vi "open_dev3.vi"(4 "ViStatus":T2, 7 "InterfaceInfo 2":T3) -> (0 "ViStatus 2":T2, 1 "drv_name":string, 2 "ModuleInfo":T1 {"DacScaleCoef" format="%#_2g"; "DacOffsetCoef" format="%#_2g"}, 3 "InterfaceInfo":T3)   [LabVIEW 2010]
uses:
  Rtusbapi.llb/3000pars.vi
  pdv_usb/wrRtusbapi.dll
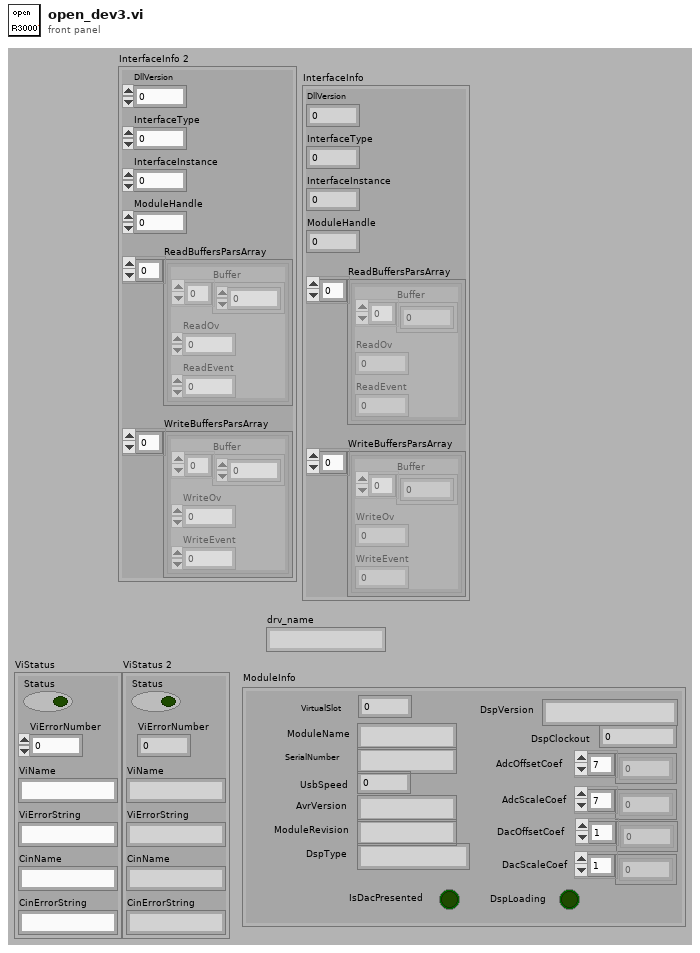
[diagram p1: front panel]
types:
  T1 = cluster{"VirtualSlot":u16, "ModuleName":string, "SerialNumber":string, "UsbSpeed":u8, "AvrVersion":string, "ModuleRevision":string, "DspType":string, "IsDacPresented":bool, "DspLoading":bool, "DspVersion":string, "DspClockout":u32, "AdcOffsetCoef":sgl[], "AdcScaleCoef":sgl[], "DacOffsetCoef":sgl[], "DacScaleCoef":sgl[]}
  T2 = cluster{"Status":bool, "ViErrorNumber":u32, "ViName":string, "ViErrorString":string, "CinName":string, "CinErrorString":string}
  T3 = cluster{"DllVersion":u32, "InterfaceType":u32, "InterfaceInstance":u32, "ModuleHandle":u32, "ReadBuffersParsArray":cluster{"Buffer":i16[], "ReadOv":u32, "ReadEvent":u32}[], "WriteBuffersParsArray":cluster{"Buffer":i16[], "WriteOv":u32, "WriteEvent":u32}[]}
  T4 = cluster{"CRC16":u16, "size":u16, "SerialNumber":string, "Name":string, "Revision":string, "DSPType":string, "IsDACPresent":u16, "DSPClockout":u32, "ADCOffset":sgl[], "ADCScale":sgl[], "DACOffset":sgl[], "DACScale":sgl[]}
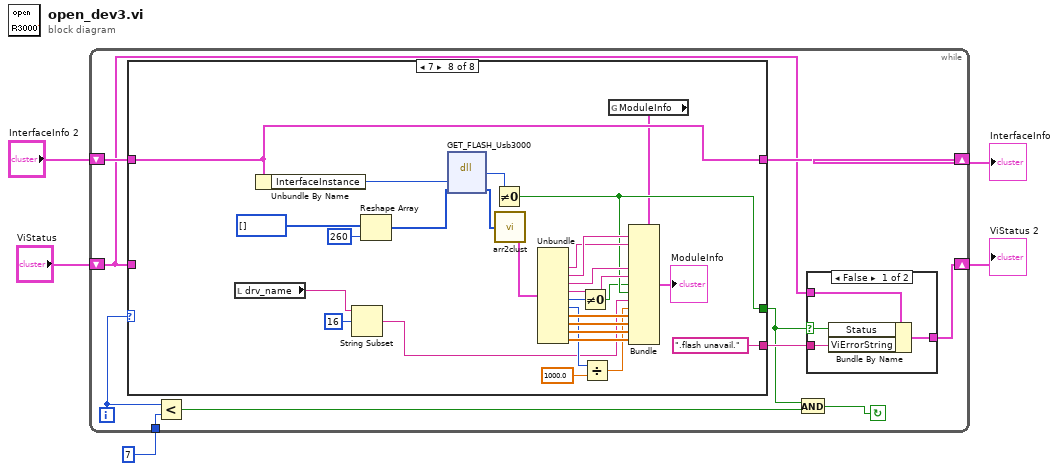
[diagram p0: block diagram]
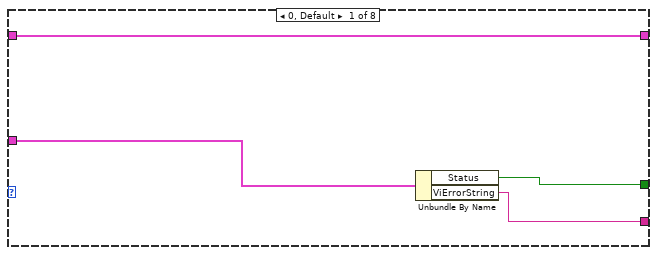
[diagram p3: hidden frame]
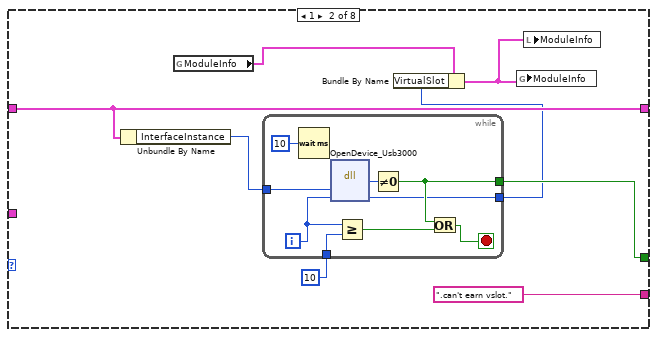
[diagram p4: hidden frame]
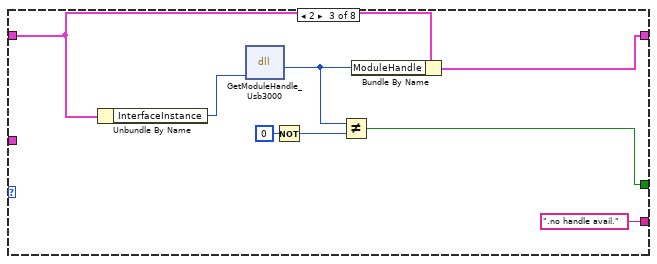
[diagram p5: hidden frame]
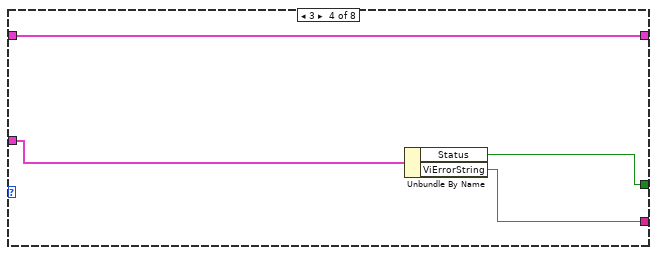
[diagram p6: hidden frame]
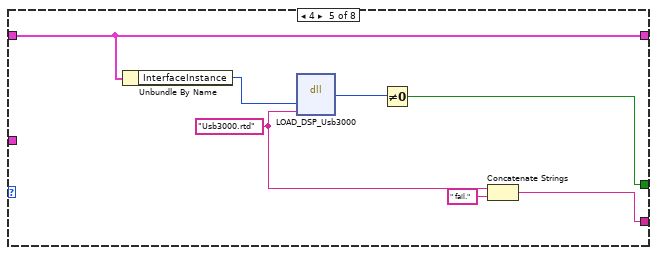
[diagram p7: hidden frame]
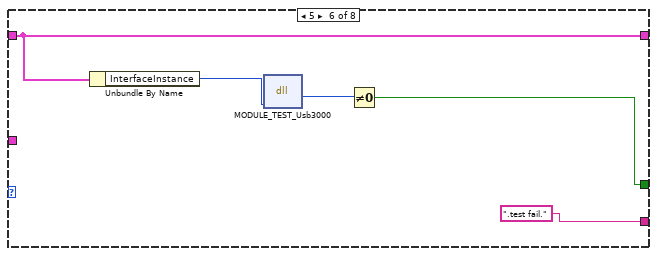
[diagram p8: hidden frame]
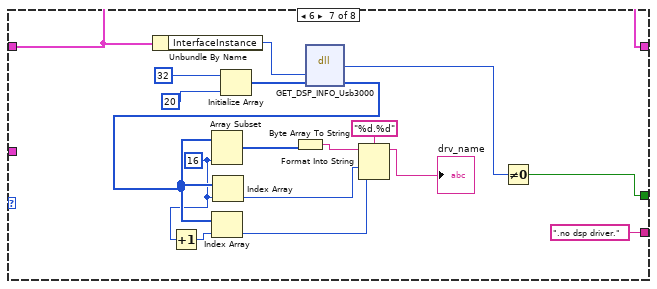
[diagram p9: hidden frame]
diagram:
  n1 = while {
    shift-right: [w14] -> w3
    shift-left: "InterfaceInfo 2" -> [w15]
    shift-right: [w12] -> w2
    shift-left: "ViStatus" -> [w13]
    tunnel: 7 ("y") -> [w6]
    i -> [w10]
    stop <- w7 continue-if-true
    n2 = case shown="7" w10 {
      tunnel: w15 -> [w24 w31 w48 w53 w60 w62 w79 w110]
      tunnel: [w24 w31 w47 w53 w60 w62 w79 w110] -> w14
      tunnel: w13 -> [w23 _ _ w51 _ _ _ _]
      tunnel: [w22 w30 w43 w52 w57 w63 w76 w96] -> w9
      tunnel: [w21 ".can't earn vslot." ("ViErrorString") ".no handle avail." ("ViErrorString") w50 w55 ".test fail." ("ViErrorString") ".no dsp driver." ("ViErrorString") ".flash unavail." ("ViErrorString")] -> w11
      frame 0, Default {
        n3 = Unbundle By Name(w23) -> ("Status"=w22:bool, "ViErrorString"=w21:string)
      }
      frame 1 {
        n4 = Unbundle By Name(w31) -> ("InterfaceInstance"=w32:u32)
        n5 = global read "3000pars.vi" "ModuleInfo"() -> (w26:T1)
        n6 = while {
          tunnel: w32 -> [w41]
          tunnel: [w37] -> w30
          tunnel: 10 -> [w38]
          tunnel: [w34] -> w27
          i -> [w39]
          stop <- w36 stop-if-true
          n7 = Wait (ms)(milliseconds to wait=u32 10) -> ()  [unwired: 1 out]
          n8 = dll-call lib="E:/Work/Andrew/Andrew_STEND/usb3k1064/pdv_usb/wrRtusbapi.dll" fn="OpenDevice_Usb3000"(w41, w39) -> (w40:i32, w34:u32)  [unwired: 4 in, 2 out]
          n9 = Greater Or Equal?(x=w39, y=w38) -> (x >= y?=w35:bool)
          n10 = Not Equal To 0?(x=w40) -> (x != 0?=w37:bool)
          n11 = Or(x=w37, y=w35) -> (x .or. y?=w36:bool)
        }
        n12 = Bundle By Name(cluster=w26, "VirtualSlot"=w27) -> (w25:T1)
        n13 = global write "3000pars.vi" "ModuleInfo"(w25) -> ()
        n14 = local write "ModuleInfo"(w25) -> ()
      }
      frame 2 {
        n15 = Unbundle By Name(w48) -> ("InterfaceInstance"=w49:u32)
        n16 = dll-call lib="E:/Work/Andrew/Andrew_STEND/usb3k1064/pdv_usb/wrRtusbapi.dll" fn="GetModuleHandle_Usb3000"(w49) -> (w46:u32)  [unwired: 4 in, 2 out]
        n17 = Not(x=u32 0 ("y")) -> (.not. x?=w44:u32)
        n18 = Not Equal?(x=w46, y=w44) -> (x != y?=w43:bool)
        n19 = Bundle By Name(cluster=w48, "ModuleHandle"=w46) -> (w47:T3)
      }
      frame 3 {
        n20 = Unbundle By Name(w51) -> ("Status"=w52:bool, "ViErrorString"=w50:string)
      }
      frame 4 {
        w56 = "Usb3000.rtd" ("input param")
        n21 = Unbundle By Name(w60) -> ("InterfaceInstance"=w59:u32)
        n22 = dll-call lib="E:/Work/Andrew/Andrew_STEND/usb3k1064/pdv_usb/wrRtusbapi.dll" fn="LOAD_DSP_Usb3000"(w59, w56) -> (w58:i32)  [unwired: 5 in, 2 out]
        n23 = Not Equal To 0?(x=w58) -> (x != 0?=w57:bool)
        n24 = Concatenate Strings(w56, " fail." ("string")) -> (w55:string)
      }
      frame 5 {
        n25 = Unbundle By Name(w62) -> ("InterfaceInstance"=w65:u32)
        n26 = dll-call lib="E:/Work/Andrew/Andrew_STEND/usb3k1064/pdv_usb/wrRtusbapi.dll" fn="MODULE_TEST_Usb3000"(w65) -> (w64:i32)  [unwired: 4 in, 2 out]
        n27 = Not Equal To 0?(x=w64) -> (x != 0?=w63:bool)
      }
      frame 6 {
        w66 = 16 ("length")
        n28 = Unbundle By Name(w79) -> ("InterfaceInstance"=w78:u32)
        n29 = Increment(x=w66) -> (x+1=w67:i32)
        n30 = Initialize Array(u8 32, 20) -> (w82:u8[])
        n31 = dll-call lib="E:/Work/Andrew/Andrew_STEND/usb3k1064/pdv_usb/wrRtusbapi.dll" fn="GET_DSP_INFO_Usb3000"(w78, w82) -> (w77:i32, w72:u8[])  [unwired: 4 in, 2 out]
        n32 = Array Subset(array=w72, length=w66) -> (w74:u8[])  [unwired: 1 in]
        n33 = Index Array(array=w72, index=w67) -> (element=w70:u8)
        n34 = Index Array(array=w72, index=w66) -> (element=w71:u8)
        n35 = Byte Array To String(unsigned byte array=w74) -> (string=w73:string)
        n36 = Format Into String(format string="%d.%d", initial string=w73, w71, w70) -> (resulting string=→"drv_name":string)  [unwired: 1 in, 1 out]
        n37 = Not Equal To 0?(x=w77) -> (x != 0?=w76:bool)
      }
      frame 7 {
        n38 = local read "drv_name"() -> (w85:string)
        n39 = Unbundle By Name(w110) -> ("InterfaceInstance"=w108:u32)
        n40 = String Subset(string=w85, offset (0)=16) -> (substring=w84:string)  [unwired: 1 in]
        n41 = Reshape Array(u8[] [] ("input param"), 260 ("dimension size")) -> (w106:u8[])
        n42 = dll-call lib="E:/Work/Andrew/Andrew_STEND/usb3k1064/pdv_usb/wrRtusbapi.dll" fn="GET_FLASH_Usb3000"(w108, w106) -> (w109:i32, w103:u8[])  [unwired: 4 in, 2 out]
        n43 = Not Equal To 0?(x=w109) -> (x != 0?=w96:bool)
        n44 = call "arr2clust.vi"("Array"=w103) -> ("Cluster"=w102:T4)
        n45 = Unbundle(w102) -> ("SerialNumber"=w99:string, "Name"=w100:string, "Revision"=w98:string, "DSPType"=w97:string, "IsDACPresent"=w91:u16, "DSPClockout"=w88:u32, "ADCOffset"=w95:sgl[], "ADCScale"=w94:sgl[], "DACOffset"=w93:sgl[], "DACScale"=w92:sgl[])  [unwired: 2 out]
        n46 = Not Equal To 0?(x=w91) -> (x != 0?=w90:bool)
        n47 = Divide(x=w88, y=1000.0) -> (x/y=w87:dbl)
        n48 = global read "3000pars.vi" "ModuleInfo"() -> (w83:T1)
        n49 = Bundle(cluster=w83, "ModuleName"=w100, "SerialNumber"=w99, "ModuleRevision"=w98, "DspType"=w97, "IsDacPresented"=w90, "DspLoading"=w96, "DspVersion"=w84, "DspClockout"=w87, "AdcOffsetCoef"=w95, "AdcScaleCoef"=w94, "DacOffsetCoef"=w93, "DacScaleCoef"=w92) -> (→"ModuleInfo":T1)  [unwired: 3 in]
      }
    }
    n50 = Less?(x=w10, y=w6) -> (x < y?=w8:bool)
    n51 = And(x=w9, y=w8) -> (x .and. y?=w7:bool)
    n52 = case shown="False" w9 {
      selector: w9 -> [w16 _]
      tunnel: w13 -> [w19 w20]
      tunnel: [w18 w20] -> w12
      tunnel: w11 -> [w17 _]
      frame False {
        n53 = Bundle By Name(cluster=w19, "Status"=w16, "ViErrorString"=w17) -> (w18:T2)
      }
      frame True {
        # "ok"
      }
    }
  }
  "InterfaceInfo" <- w3
  "ViStatus 2" <- w2
